vi "Read Line.vi"(8 "error in (no error)":errorcluster) -> (0 "error out":errorcluster, 1 "Line length":i32, 2 "Line":string)   [LabVIEW 2017]
uses:
  Variables/MyRIO Lidar Class Data.vi
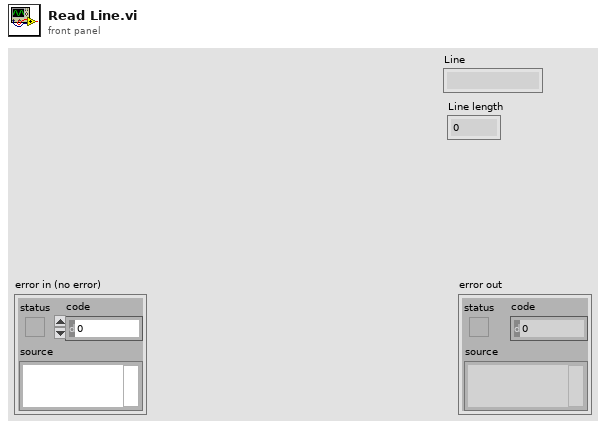
[diagram p1: front panel]
types:
  T1 = cluster{"Shared library path":path, "File Descriptor":i32}
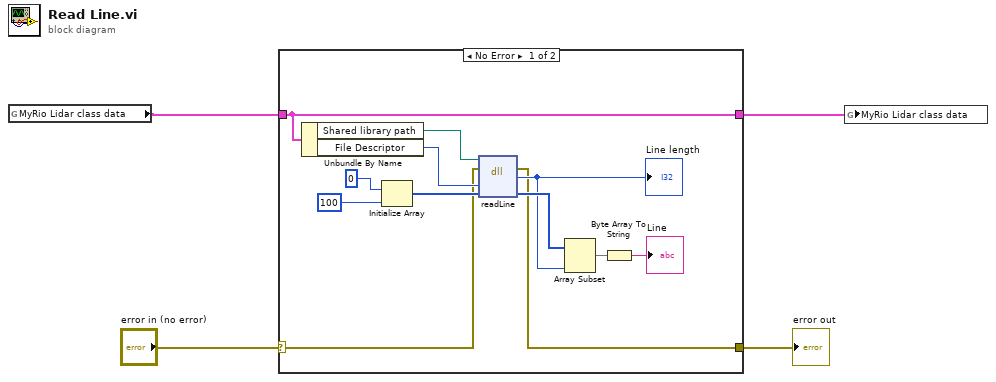
[diagram p0: block diagram]
diagram:
  n1 = global read "MyRIO Lidar Class Data.vi" "MyRio Lidar class data"() -> (w2:T1)
  n2 = case shown="No Error" "error in (no error)" {
    selector: "error in (no error)" -> [w6 w18]
    tunnel: [w5 w18] -> w3
    tunnel: w2 -> [w7 w17]
    tunnel: [w7 w17] -> w1
    frame No Error {
      n3 = Unbundle By Name(w7) -> ("Shared library path"=w9:path, "File Descriptor"=w8:i32)
      n4 = Initialize Array(u8 0 ("element"), 100 ("dimension size")) -> (w16:u8[])
      n5 = dll-call lib="?" fn="readLine"(path in=w9, error in=w6, "fd"=w8, "buff"=w16) -> (error out=w5:errorcluster, "return type"=w10:i32, "buff"=w13:u8[])  [unwired: 2 in, 1 out]
      "Line length" <- w10
      n6 = Array Subset(array=w13, length=w10) -> (w12:u8[])  [unwired: 1 in]
      n7 = Byte Array To String(unsigned byte array=w12) -> (string=→"Line":string)
    }
    frame Error {
    }
  }
  "error out" <- w3
  n8 = global write "MyRIO Lidar Class Data.vi" "MyRio Lidar class data"(w1) -> ()
